vi "Read Protocol.vi"(8 "error in (no error)":errorcluster, 11 "Subscription in":refnum<class "Subscription.lvclass">) -> (0 "error out":errorcluster, 2 "Subscription Protocol":T1, 3 "Subscription out":refnum<class "Subscription.lvclass">)   [LabVIEW 2015, in "NI_AWS_SNS.lvlib" / "Subscription.lvclass"]
uses:
  Subscription.lvclass
  Subscription Protocol.ctl
  Subscription.lvclass/Subscription.ctl
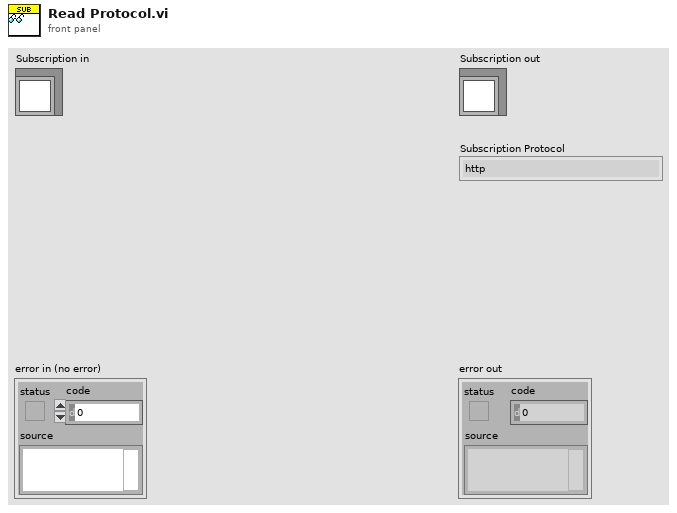
[diagram p1: front panel]
types:
  T1 = typedef "NI_AWS_SNS.lvlib/Subscription.lvclass/Subscription Protocol.ctl" = enum16{"http", "https", "email", "email-json", "sms", "sqs", "application", "lambda"}
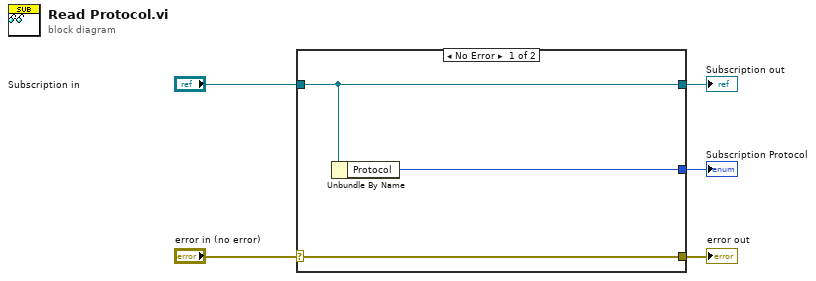
[diagram p0: block diagram]
diagram:
  n1 = case shown="No Error" "error in (no error)" {
    selector: "error in (no error)" -> [w8 w9]
    tunnel: [w8 w9] -> w4
    tunnel: [w7 w10] -> w2
    tunnel: "Subscription in" -> [w7 w10]
    tunnel: [w6 _] -> w1
    frame No Error {
      n2 = Unbundle By Name(w7) -> ("Protocol"=w6:T1)
    }
    frame Error {
    }
  }
  "error out" <- w4
  "Subscription out" <- w2
  "Subscription Protocol" <- w1
